vi "CarWashTestcase.vi"(11 "error in":errorcluster) -> (15 "error out":errorcluster)   [LabVIEW 2016]
uses:
  <vilib>/addons/_JKI Toolkits/Caraya/classes/Test/Test.lvclass
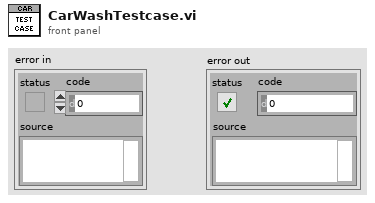
[diagram p1: front panel]
types:
  T1 = cluster{"Wash Option":string, "Car Position":u8, "Elapsed Time":dbl}[]
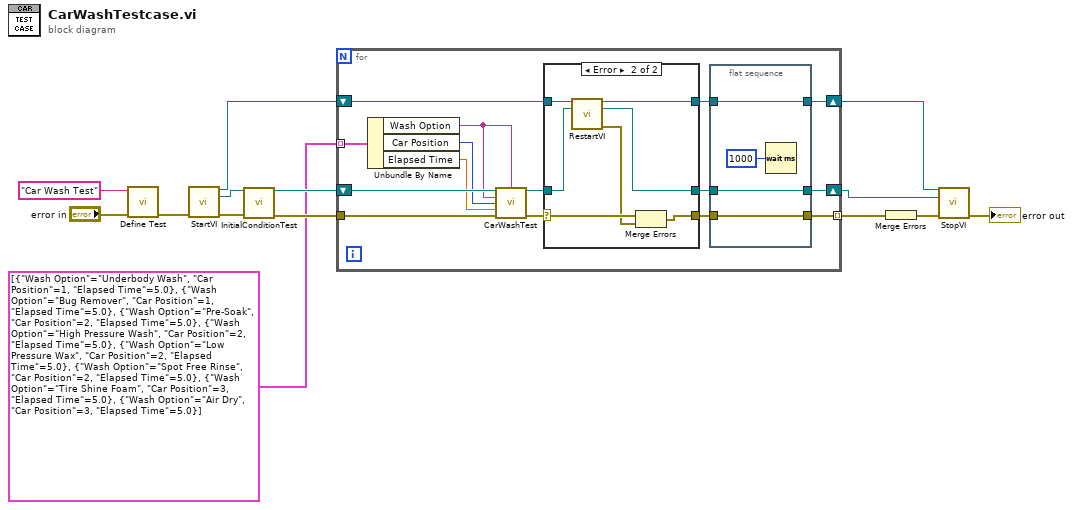
[diagram p0: block diagram]
diagram:
  n1 = call <vilib>:"Define Test.vi"("error in (no error)"="error in", "Label (VI Title)"="Car Wash Test" ("Label")) -> ("error out"=w6:errorcluster)  [unwired: 9 in]
  n2 = call "StartVI.vi"("error in"=w6) -> ("Application Ref out"=w2:refnum<vi>, "VI Reference"=w4:refnum<vi>, "error out"=w14:errorcluster)  [unwired: 12 in]
  n3 = call "InitialConditionTest.vi"("VI Reference In"=w4, "error in"=w14) -> ("VI Reference Out"=w12:refnum<vi>, "error out"=w13:errorcluster)  [unwired: 12 in]
  n4 = for {
    shift-right: [w17] -> w3
    shift-left: w12 -> [w28]
    tunnel: T1 [{"Wash Option"="Underbody Wash", "Car Position"=1, "Elapsed Time"=5.0}, {"Wash Option"="Bug Remover", "Car Position"=1, "Elapsed Time"=5.0}, {"Wash Option"="Pre-Soak", "Car Position"=2, "Elapsed Time"=5.0}, {"Wash Option"="High Pressure Wash", "Car Position"=2, "Elapsed Time"=5.0}, {"Wash Option"="Low Pressure Wax", "Car Position"=2, "Elapsed Time"=5.0}, {"Wash Option"="Spot Free Rinse", "Car Position"=2, "Elapsed Time"=5.0}, {"Wash Option"="Tire Shine Foam", "Car Position"=3, "Elapsed Time"=5.0}, {"Wash Option"="Air Dry", "Car Position"=3, "Elapsed Time"=5.0}] -> [w27] mode=indexing
    tunnel: w13 -> [w29]
    tunnel: [w20] -> w9 mode=indexing
    shift-right: [w16] -> w1
    shift-left: w2 -> [w21]
    n5 = Unbundle By Name(w27) -> ("Wash Option"=w24:string, "Car Position"=w26:u8, "Elapsed Time"=w25:dbl)
    n6 = call "CarWashTest.vi"("VI Reference In"=w28, "Label"=w24, "Wash Option"=w24, "Car Position"=w26, "Elapsed Time"=w25, "error in"=w29) -> ("VI Reference Out"=w22:refnum<vi>, "error out"=w23:errorcluster)  [unwired: 8 in]
    n7 = case shown="Error" w23 {
      selector: w23 -> [w35 w43]
      tunnel: [w35 w42] -> w19
      tunnel: w22 -> [w36 w39]
      tunnel: [w36 w40] -> w18
      tunnel: [w34 w37] -> w15
      tunnel: w21 -> [w34 w38]
      frame No Error {
      }
      frame Error {
        n8 = call "RestartVI.vi"("Application Ref in"=w38, "VI in"=w39) -> ("Application Ref out"=w37:refnum<vi>, "VI out"=w40:refnum<vi>, "error out"=w41:errorcluster)  [unwired: 11 in]
        n9 = Merge Errors(w43, w41) -> (w42:errorcluster)
      }
    }
    n10 = flat-sequence {
      tunnel: [w33] -> w20
      tunnel: w19 -> [w33]
      tunnel: w18 -> [w32]
      tunnel: [w32] -> w17
      tunnel: [w31] -> w16
      tunnel: w15 -> [w31]
      frame #0 {
        n11 = Wait (ms)(milliseconds to wait=u32 1000) -> ()  [unwired: 1 out]
      }
    }
  }
  n12 = Merge Errors(w9) -> (w11:errorcluster)
  n13 = call "StopVI.vi"("Application Ref in"=w1, "VI in"=w3, "error in (no error)"=w11) -> ("error out"=→"error out":errorcluster)  [unwired: 12 in]
